vi "FreeCOM.vi"() -> ()   [LabVIEW 2012]
uses:
  <vilib>/Instr/_visa.llb/VISA Configure Serial Port (Serial Instr).vi
panel:
  in  "Enable":bool=TRUE
  out "Ram":string
  in  "保存数据":bool
  in  "清空接收区":bool
  in  "清空波形区":bool
  in  "清空计数":bool
  out "RX":dbl
  out "TX":dbl
  in  "换行":bool
  in  "send":bool
  in  "发送区":string
  out "串口波形图":dbl(graph)
  out "接收区":string
  in  "端口号":u16(ring) caption="Port" items=["COM1", "COM2", "COM3", "COM4", "COM5"]
  in  "波特率":u16(ring) caption="Baud" items=["9600", "115200"]
  out "串口状态":bool
  in  "exit":bool
  in  "open":bool
  # "Count"
  # "Config"
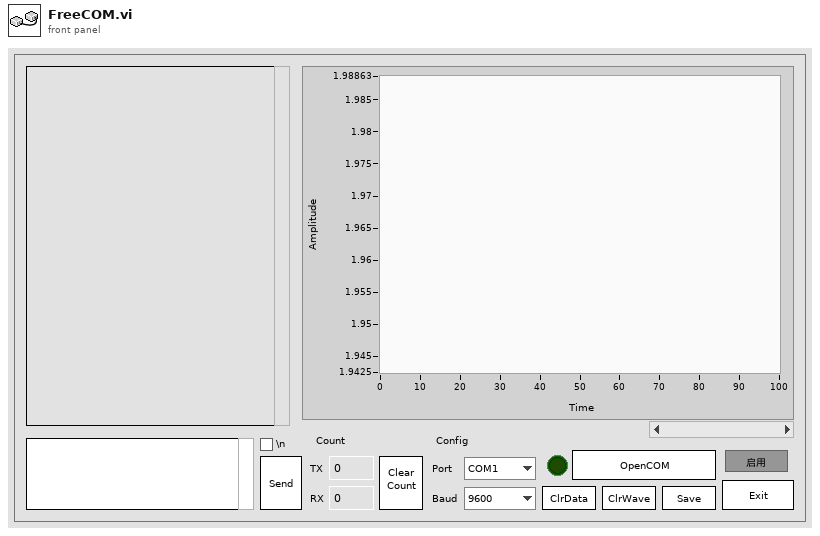
[diagram p1: front panel]
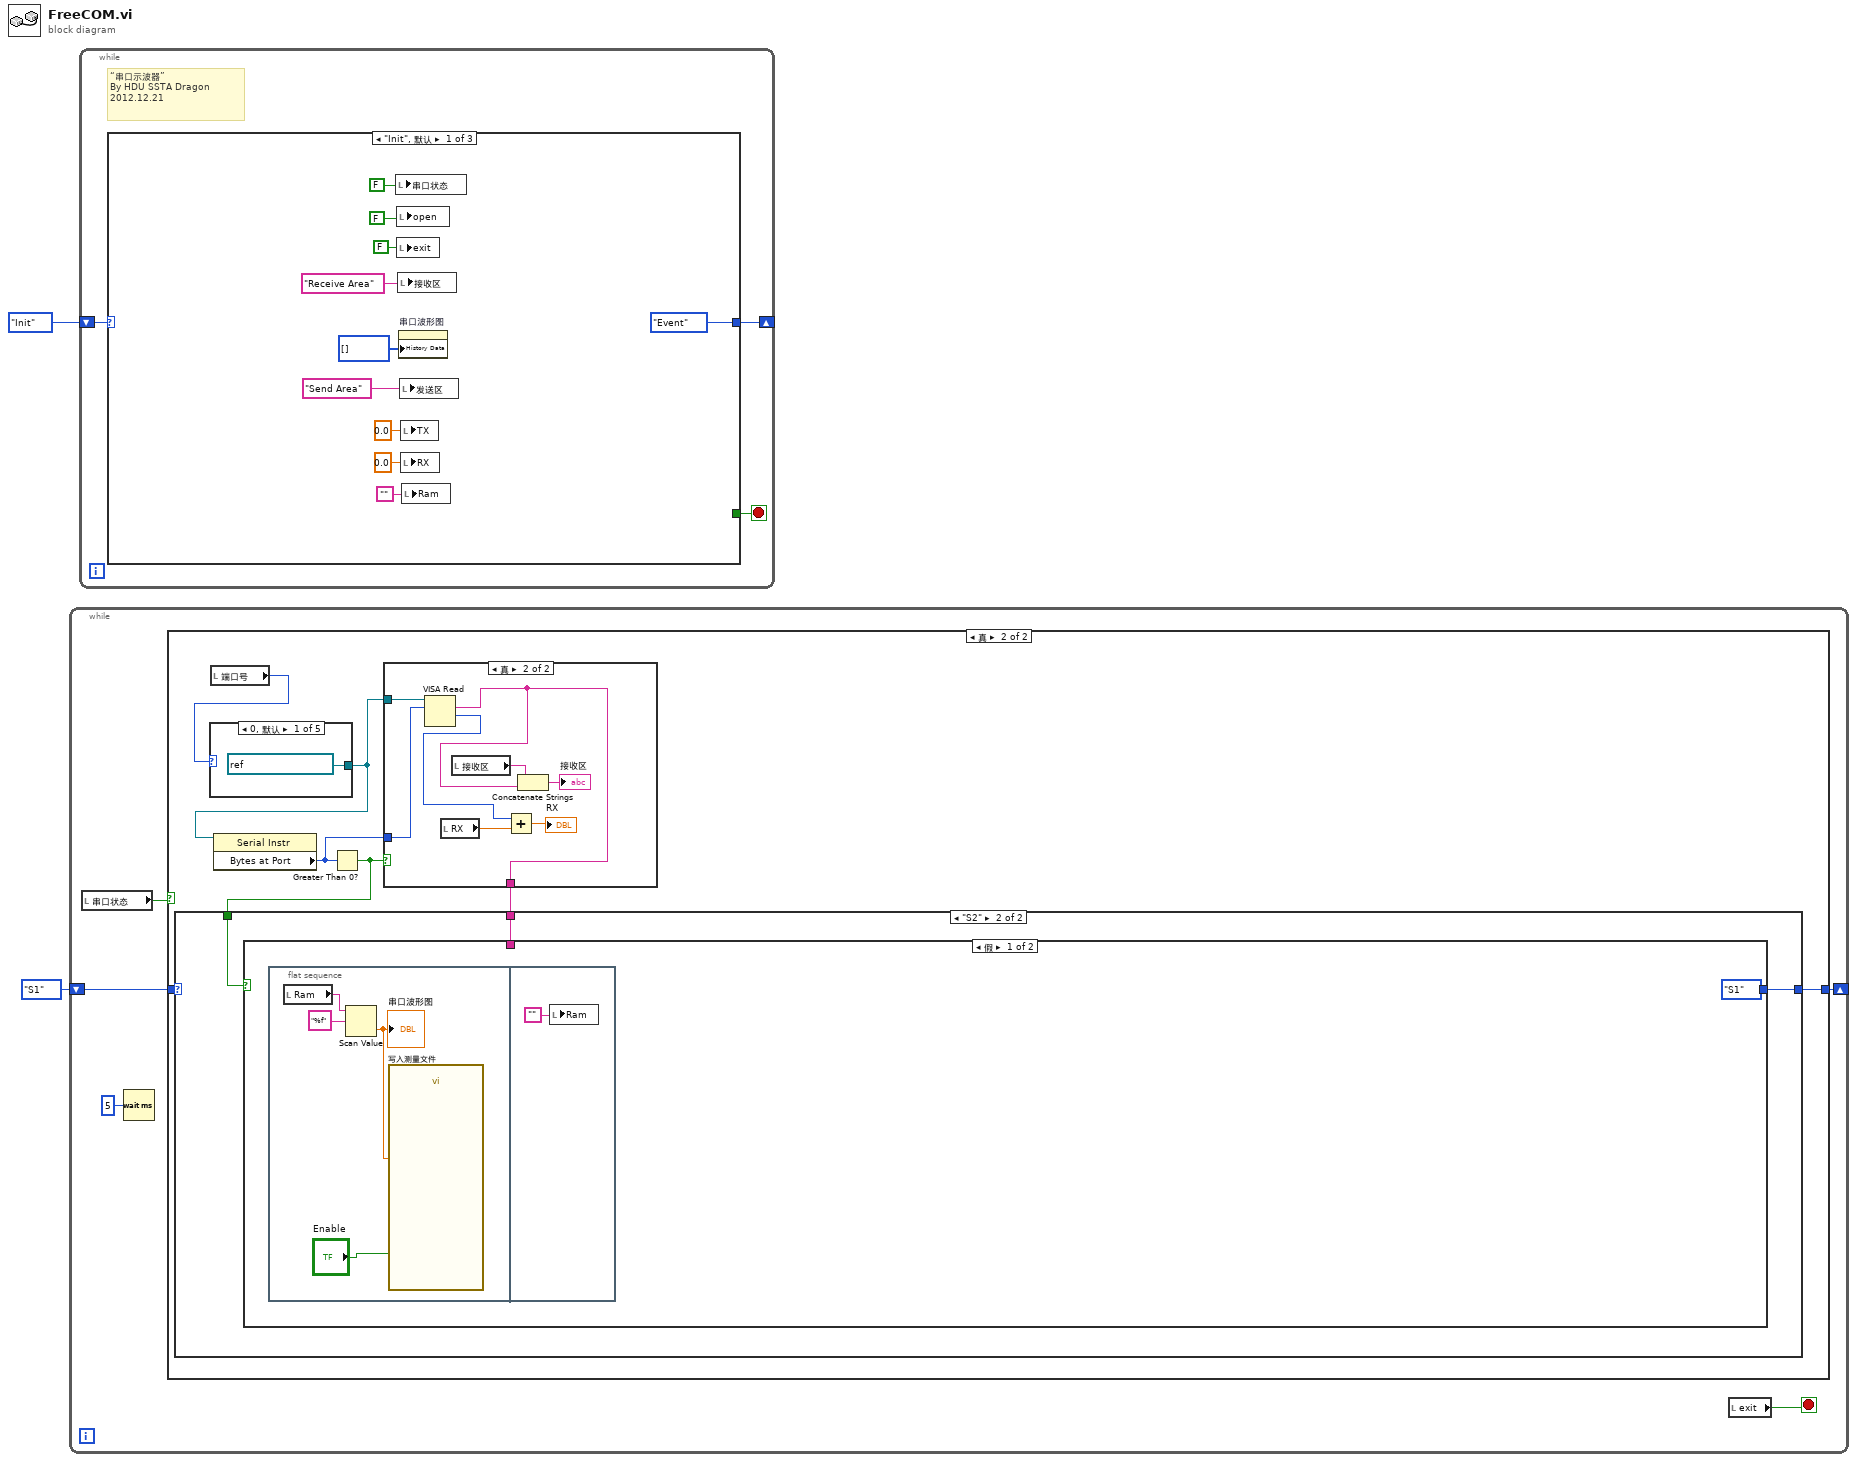
[diagram p0: block diagram]
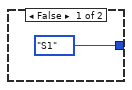
[diagram p2: hidden frame]
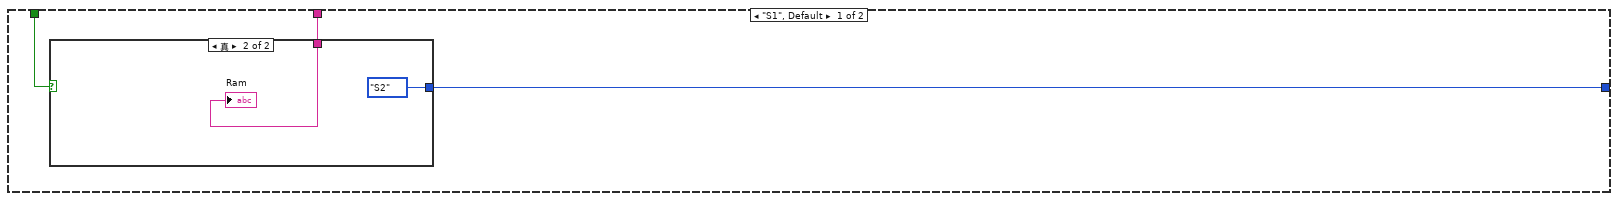
[diagram p3: hidden frame]
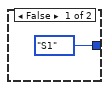
[diagram p4: hidden frame]
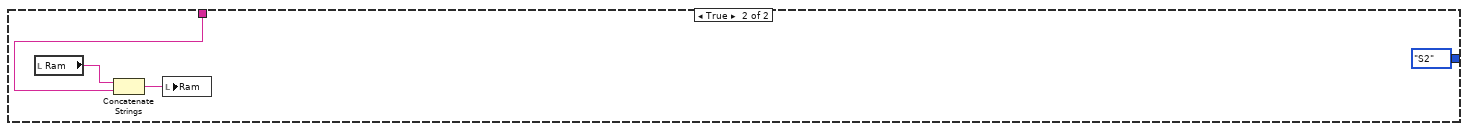
[diagram p5: hidden frame]
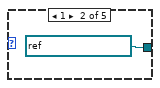
[diagram p7: hidden frame]
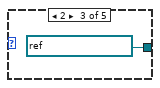
[diagram p8: hidden frame]
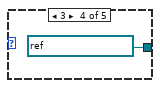
[diagram p9: hidden frame]
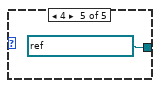
[diagram p10: hidden frame]
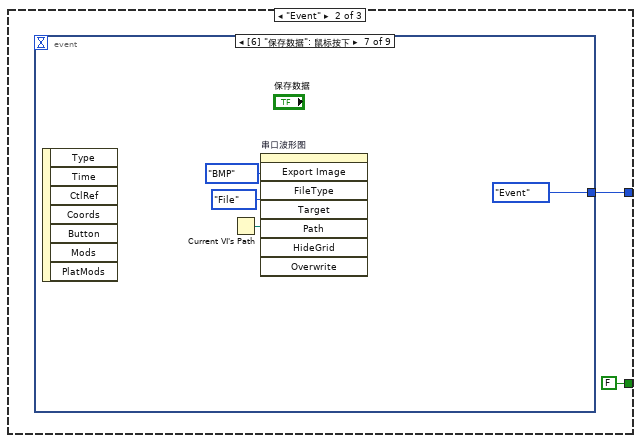
[diagram p11: hidden frame]
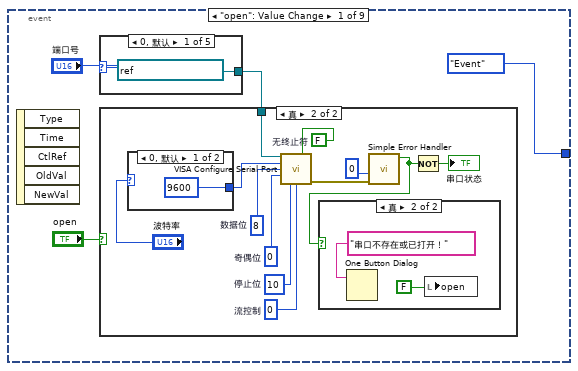
[diagram p12: hidden frame]
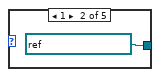
[diagram p13: hidden frame]
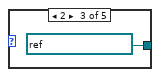
[diagram p14: hidden frame]
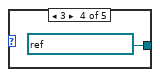
[diagram p15: hidden frame]
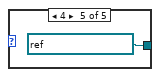
[diagram p16: hidden frame]
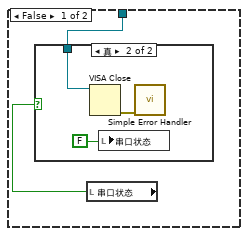
[diagram p17: hidden frame]
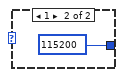
[diagram p20: hidden frame]
diagram:
  n1 = while {
    shift-right: [w5] -> _
    shift-left: enum16{"S1", "S2"}."S1" -> [w6]
    stop <- w3 stop-if-true
    n2 = local read "串口状态"() -> (w4:bool)
    n3 = Wait (ms)(milliseconds to wait=u32 5 ("等待时间（毫秒）")) -> ()  [unwired: 1 out]
    n4 = case shown="真" w4 {
      tunnel: w6 -> [_ w12]
      tunnel: [enum16{"S1", "S2"}."S1" w9] -> w5
      frame False {
      }
      frame True {
        n5 = local read "端口号"() -> (w15:u16)
        n6 = case shown="0, 默认" w15 {
          tunnel: [refnum<visa-resource-name> "ASRL1::INSTR" ("VISA resource name") refnum<visa-resource-name> "ASRL2::INSTR" ("VISA resource name") refnum<visa-resource-name> "ASRL3::INSTR" ("VISA resource name") refnum<visa-resource-name> "ASRL4::INSTR" ("VISA resource name") refnum<visa-resource-name> "ASRL5::INSTR" ("VISA resource name")] -> w14
          frame 0, Default {
          }
          frame 1 {
          }
          frame 2 {
          }
          frame 3 {
          }
          frame 4 {
          }
        }
        n7 = property class="Serial Instr"(reference=w14) -> ("Bytes at Port"=w13:u32)  [unwired: 1 in, 2 out]
        n8 = Greater Than 0?(x=w13) -> (x > 0?=w11:bool)
        n9 = case shown="真" w11 {
          tunnel: w14 -> [_ w42]
          tunnel: w13 -> [_ w37]
          tunnel: [_ w36] -> w10
          frame False {
          }
          frame True {
            n10 = VISA Read(VISA resource name=w42, byte count=w37) -> (read buffer=w36:string, return count=w35:u32)  [unwired: 1 in, 2 out]
            n11 = local read "RX"() -> (w39:dbl)
            n12 = local read "接收区"() -> (w40:string)
            n13 = Add(x=w35, y=w39) -> (x+y=→"RX":dbl)
            n14 = Concatenate Strings(w40, w36) -> (→"接收区":string)
          }
        }
        n15 = case shown="\"S2\"" w12 {
          tunnel: w11 -> [w18 w24]
          tunnel: w10 -> [w17 w22]
          tunnel: [w16 w23] -> w9
          frame "S1", Default {
            n16 = case shown="真" w18 {
              tunnel: w17 -> [_ w21]
              tunnel: [enum16{"S1", "S2"}."S1" enum16{"S1", "S2"}."S2"] -> w16
              frame False {
              }
              frame True {
                "Ram" <- w21
              }
            }
          }
          frame "S2" {
            n17 = case shown="假" w24 {
              tunnel: [enum16{"S1", "S2"}."S1" enum16{"S1", "S2"}."S2"] -> w23
              tunnel: w22 -> [_ w31]
              frame False {
                n18 = flat-sequence {
                  frame #0 {
                    n19 = local read "Ram"() -> (w26:string)
                    n20 = Scan Value(string=w26, format string="%f" ("格式字符串")) -> (value=w27:dbl)  [unwired: 1 in, 1 out]
                    "串口波形图" <- w27
                    n21 = call "写入测量文件"("Signals"=w27, "Enable"="Enable") -> ()  [unwired: 15 in, 3 out]
                  }
                  frame #1 {
                    n22 = local write "Ram"("") -> ()
                  }
                }
              }
              frame True {
                n23 = local read "Ram"() -> (w32:string)
                n24 = Concatenate Strings(w32, w31) -> (w33:string)
                n25 = local write "Ram"(w33) -> ()
              }
            }
          }
        }
      }
    }
    n26 = local read "exit"() -> (w3:bool)
  }
  n27 = while {
    shift-right: [w48] -> _
    shift-left: enum16{"Init", "Event", "Exit"}."Init" -> [w49]
    stop <- w50 stop-if-true
    # "“串口示波器”\nBy HDU SSTA Dragon\n2012.12.21"
    n28 = case shown="\"Init\", 默认" w49 {
      tunnel: [_ FALSE TRUE] -> w50
      tunnel: [enum16{"Init", "Event", "Exit"}."Event" w61 enum16{"Init", "Event", "Exit"}."Exit"] -> w48
      frame "Init", Default {
        n29 = local write "串口状态"(FALSE) -> ()
        n30 = local write "open"(FALSE) -> ()
        n31 = local write "exit"(FALSE ("exit")) -> ()
        n32 = local write "接收区"("Receive Area") -> ()
        n33 = property on="串口波形图" class="WFChart (严格)"("History Data"=u8[] [] ("历史数据")) -> ()  [unwired: 2 in, 2 out]
        n34 = local write "发送区"("Send Area" ("发送区")) -> ()
        n35 = local write "TX"(0.0 ("TX")) -> ()
        n36 = local write "RX"(0.0 ("RX")) -> ()
        n37 = local write "Ram"("") -> ()
      }
      frame "Event" {
        n38 = event shown="[6] \"保存数据\": 鼠标按下" {
          selector: _ -> [_ _ _ _ _ _ _ _ _]
          dyn-events: _ -> [_ _ _ _ _ _ _ _ _]
          timeout: _ -> [_ _ _ _ _ _ _ _ _]
          tunnel: [enum16{"Init", "Event", "Exit"}."Event" enum16{"Init", "Event", "Exit"}."Event" enum16{"Init", "Event", "Exit"}."Event" enum16{"Init", "Event", "Exit"}."Event" enum16{"Init", "Event", "Exit"}."Event" enum16{"Init", "Event", "Exit"}."Event" enum16{"Init", "Event", "Exit"}."Event" enum16{"Init", "Event", "Exit"}."Event" enum16{"Init", "Event", "Exit"}."Exit"] -> w61
          event "open": Value Change {
            n39 = event-data() -> ()  [unwired: 1 in, 5 out]
            n40 = case shown="0, 默认" "端口号" {
              tunnel: [refnum<visa-resource-name> "ASRL1::INSTR" ("VISA resource name") refnum<visa-resource-name> "ASRL2::INSTR" ("VISA resource name") refnum<visa-resource-name> "ASRL3::INSTR" ("VISA resource name") refnum<visa-resource-name> "ASRL4::INSTR" ("VISA resource name") refnum<visa-resource-name> "ASRL5::INSTR" ("VISA resource name")] -> w65
              frame 0, Default {
              }
              frame 1 {
              }
              frame 2 {
              }
              frame 3 {
              }
              frame 4 {
              }
            }
            n41 = case shown="真" "open" {
              tunnel: w65 -> [w73 w78]
              frame False {
                n42 = local read "串口状态"() -> (w72:bool)
                n43 = case shown="真" w72 {
                  tunnel: w73 -> [_ w74]
                  frame False {
                  }
                  frame True {
                    n44 = VISA Close(VISA resource name=w74) -> (error out=w76:errorcluster)  [unwired: 1 in]
                    n45 = local write "串口状态"(FALSE) -> ()
                    n46 = call <vilib>:"Simple Error Handler.vi"("error in (no error)"=w76) -> ()  [unwired: 4 in, 5 out]
                  }
                }
              }
              frame True {
                w79 = FALSE  # 无终止符
                w86 = u16 0  # 流控制
                w85 = u16 10  # 停止位
                w84 = u8 0  # 奇偶位
                w83 = u16 8  # 数据位
                n47 = case shown="0, 默认" "波特率" {
                  tunnel: [u32 9600 u32 115200] -> w82
                  frame 0, Default {
                  }
                  frame 1 {
                  }
                }
                n48 = call-poly "VISA Configure Serial Port"("VISA resource name"=w78, "Enable Termination\nChar (T)"=w79, "baud rate (9600)"=w82, "data bits (8)"=w83, "parity (0:none)"=w84, "stop bits (10: 1 bit)"=w85, "flow control (0:none)"=w86) -> ("error out"=w87:errorcluster)  [unwired: 7 in, 1 out]
                n49 = call <vilib>:"Simple Error Handler.vi"("type of dialog (OK msg:1)"=0, "error in (no error)"=w87) -> ("error?"=w80:bool)  [unwired: 3 in, 4 out]
                n50 = case shown="真" w80 {
                  frame False {
                  }
                  frame True {
                    n51 = One Button Dialog(message="串口不存在或已打开！") -> ()  [unwired: 1 in, 1 out]
                    n52 = local write "open"(FALSE) -> ()
                  }
                }
                n53 = Not(x=w80) -> (.not. x?=→"串口状态":bool)
              }
            }
          }
          event "端口号", "波特率": Value Change {
            n54 = event-data() -> ("OldVal"=w94:u16)  [unwired: 1 in, 4 out]
            n55 = local read "串口状态"() -> (w95:bool)
            n56 = case shown="真" w95 {
              tunnel: w94 -> [_ w96]
              frame False {
              }
              frame True {
                n57 = flat-sequence {
                  tunnel: w96 -> [w101]
                  frame #0 {
                    n58 = case shown="0, 默认" w101 {
                      tunnel: [refnum<visa-resource-name> "ASRL1::INSTR" ("VISA resource name") refnum<visa-resource-name> "ASRL2::INSTR" ("VISA resource name") refnum<visa-resource-name> "ASRL3::INSTR" ("VISA resource name") refnum<visa-resource-name> "ASRL4::INSTR" ("VISA resource name") refnum<visa-resource-name> "ASRL5::INSTR" ("VISA resource name")] -> w98
                      frame 0, Default {
                      }
                      frame 1 {
                      }
                      frame 2 {
                      }
                      frame 3 {
                      }
                      frame 4 {
                      }
                    }
                    n59 = VISA Close(VISA resource name=w98) -> (error out=w100:errorcluster)  [unwired: 1 in]
                    n60 = call <vilib>:"Simple Error Handler.vi"("error in (no error)"=w100) -> ()  [unwired: 4 in, 5 out]
                    n61 = local write "串口状态"(FALSE) -> ()
                    n62 = local write "open"(FALSE ("open")) -> ()
                  }
                }
              }
            }
          }
          event "send": Mouse Down {
            n63 = event-data() -> ()  [unwired: 1 in, 7 out]
            n64 = local read "串口状态"() -> (w108:bool)
            n65 = case shown="真" w108 {
              frame False {
              }
              frame True {
                n66 = local read "端口号"() -> (w118:u16)
                n67 = case shown="真" "换行" {
                  tunnel: [_ "\r"] -> w116
                  tunnel: [_ "\n"] -> w115
                  frame False {
                  }
                  frame True {
                  }
                }
                n68 = case shown="0, 默认" w118 {
                  tunnel: [refnum<visa-resource-name> "ASRL1::INSTR" ("VISA resource name") refnum<visa-resource-name> "ASRL2::INSTR" ("VISA resource name") refnum<visa-resource-name> "ASRL3::INSTR" ("VISA resource name") refnum<visa-resource-name> "ASRL4::INSTR" ("VISA resource name") refnum<visa-resource-name> "ASRL5::INSTR" ("VISA resource name")] -> w117
                  frame 0, Default {
                  }
                  frame 1 {
                  }
                  frame 2 {
                  }
                  frame 3 {
                  }
                  frame 4 {
                  }
                }
                n69 = Concatenate Strings("发送区", w116, w115) -> (w112:string)
                n70 = local read "TX"() -> (w111:dbl)
                n71 = VISA Write(VISA resource name=w117, write buffer=w112) -> (return count=w109:u32)  [unwired: 1 in, 2 out]
                n72 = Add(x=w109, y=w111) -> (x+y=→"TX":dbl)
              }
            }
          }
          event "清空计数": Mouse Down {
            n73 = event-data() -> ()  [unwired: 1 in, 7 out]
            n74 = local write "RX"(0.0 ("RX")) -> ()
            n75 = local write "TX"(0.0 ("TX")) -> ()
          }
          event "清空接收区": Mouse Down {
            n76 = event-data() -> ()  [unwired: 1 in, 7 out]
            n77 = local write "接收区"("") -> ()
          }
          event "清空波形区": Mouse Down {
            n78 = event-data() -> ()  [unwired: 1 in, 7 out]
            n79 = property on="串口波形图" class="WFChart (严格)"("History Data"=u8[] [] ("历史数据")) -> ()  [unwired: 2 in, 2 out]
          }
          event "保存数据": Mouse Down {
            n80 = event-data() -> ()  [unwired: 1 in, 7 out]
            n81 = Current VI's Path() -> (path=w133:path)
            n82 = invoke on="串口波形图" class="WFChart (严格)" method="Export Image"("FileType"=enum32{"BMP", "EPS", "EMF", "PICT"}."BMP" ("文件类型"), "Target"=enum32{"File", "Clipboard"}."File" ("目标"), "Path"=w133) -> ()  [unwired: 5 in, 8 out]
          }
          event Menu Selection (User) {
            n83 = event-data() -> ("ItemTag"=w140:string)  [unwired: 1 in, 5 out]
            n84 = Equal?(x="ABOUT", y=w140) -> (x = y?=w141:bool)
            n85 = Equal?(x="USE", y=w140) -> (x = y?=w142:bool)
            n86 = case shown="真" w142 {
              frame False {
              }
              frame True {
                n87 = One Button Dialog(message="“串口示波器”\n保存的波形图像bmp在vi当前目录中" ("Message")) -> ()  [unwired: 1 in, 1 out]
              }
            }
            n88 = case shown="真" w141 {
              frame False {
              }
              frame True {
                n89 = One Button Dialog(message="By HDU SSTA Dragon\nhlimapla@gmail.com\n comm demo for cjl" ("Message")) -> ()  [unwired: 1 in, 1 out]
              }
            }
          }
          event "exit": Value Change {
            n90 = event-data() -> ()  [unwired: 1 in, 5 out]
            n91 = local read "串口状态"() -> (w148:bool)
            n92 = local read "端口号"() -> (w146:u16)
            n93 = case shown="0, 默认" w146 {
              tunnel: [refnum<visa-resource-name> "ASRL1::INSTR" ("VISA resource name") refnum<visa-resource-name> "ASRL2::INSTR" ("VISA resource name") refnum<visa-resource-name> "ASRL3::INSTR" ("VISA resource name") refnum<visa-resource-name> "ASRL4::INSTR" ("VISA resource name") refnum<visa-resource-name> "ASRL5::INSTR" ("VISA resource name")] -> w147
              frame 0, Default {
              }
              frame 1 {
              }
              frame 2 {
              }
              frame 3 {
              }
              frame 4 {
              }
            }
            n94 = case shown="真" w148 {
              tunnel: w147 -> [_ w157]
              frame False {
              }
              frame True {
                n95 = VISA Close(VISA resource name=w157) -> (error out=w156:errorcluster)  [unwired: 1 in]
                n96 = local write "串口状态"(FALSE) -> ()
                n97 = local write "open"(FALSE) -> ()
                n98 = call <vilib>:"Simple Error Handler.vi"("error in (no error)"=w156) -> ()  [unwired: 4 in, 5 out]
              }
            }
          }
        }
      }
      frame "Exit" {
      }
    }
  }
